vi "数组簇.vi"() -> ()   [LabVIEW 2014]
panel:
  out "布尔 2":bool
  out "数值":dbl
  in  "布尔":bool
  in  "簇":cluster{"数值":dbl, "布尔":bool, "字符串":string}
  out "元素":dbl
  in  "(列) 2":i32
  in  "(行)":i32
  out "大小":i32[](array[numeric])
  in  "数组":dbl[][](array[numeric])
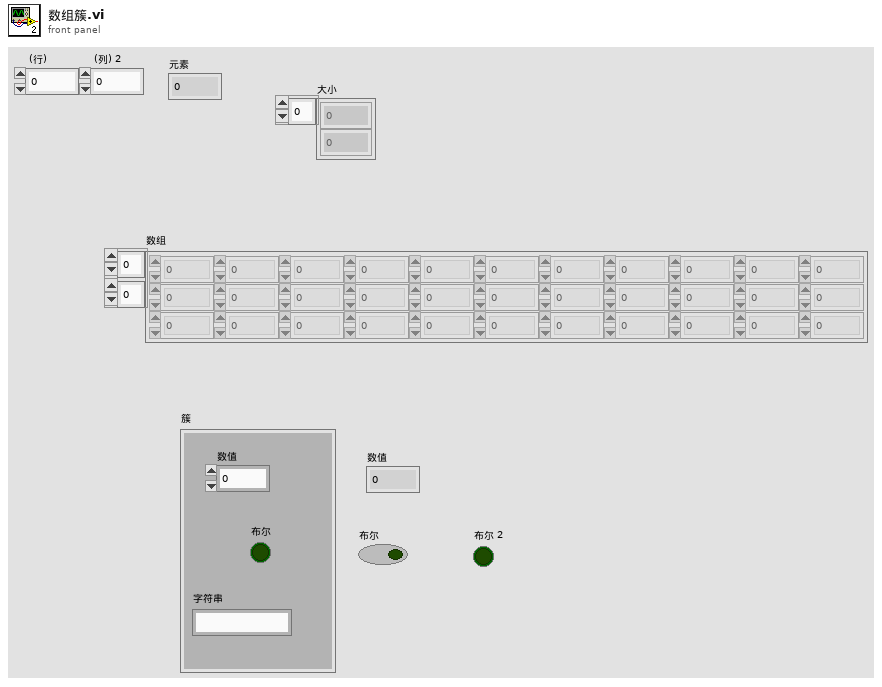
[diagram p1: front panel]
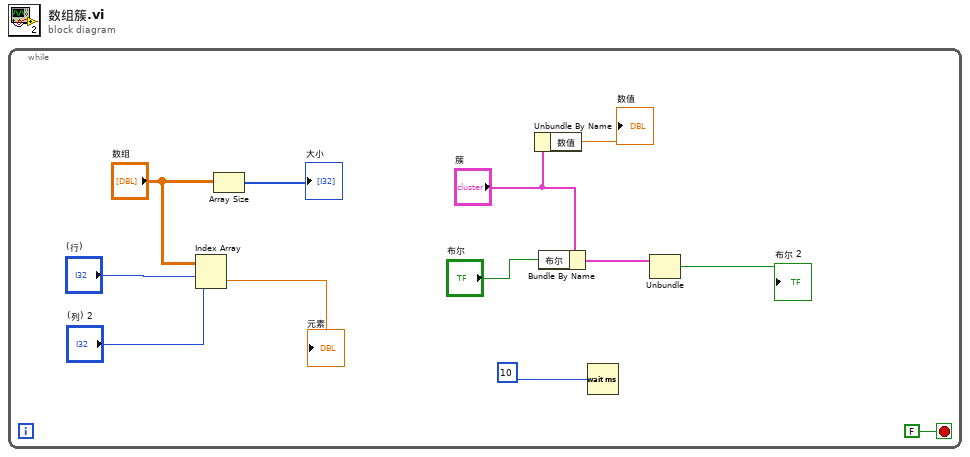
[diagram p0: block diagram]
diagram:
  n1 = while {
    stop <- FALSE stop-if-true
    n2 = Index Array(array="数组", index (row)="(行)", index (col)="(列) 2") -> (element=→"元素":dbl)
    n3 = Array Size(array="数组") -> (size(s)=→"大小":i32[])
    n4 = Unbundle By Name("簇") -> ("数值"=→"数值":dbl)
    n5 = Bundle By Name(cluster="簇", "布尔"="布尔") -> (w4:cluster{"数值":dbl, "布尔":bool, "字符串":string})
    n6 = Wait (ms)(milliseconds to wait=u32 10 ("毫秒计时值")) -> ()  [unwired: 1 out]
    n7 = Unbundle(w4) -> ("布尔"=→"布尔 2":bool)  [unwired: 2 out]
  }
